vi "iRobot Poll Sensor Group 4.vi"(8 "error in":errorcluster, 11 "UART port in":T4) -> (0 "error out":errorcluster, 1 "Timed Out?":bool, 2 "Sensor Group 4":T1, 3 "UART port out":T4)   [LabVIEW 2010]
doc: "Poll the iRobot for Sensor Group 4; blocks until response is received, or the operation has timed out.\n\nThis VI both writes to AND reads from the serial port\n<b>NOTE</b>: This should not be used in a loop if other serial reading or writing VIs are called in parallel loops."
uses:
  UART/UART Port Type.ctl
  Sensor Controls/iRobot Sensor Group 4.ctl
  Sensor Controls/iRobot Cargo Bay Digital Inputs.ctl
  Sensor Controls/iRobot Charging Sources Available.ctl
  Open Interface Controls/iRobot Sensor ID.ctl
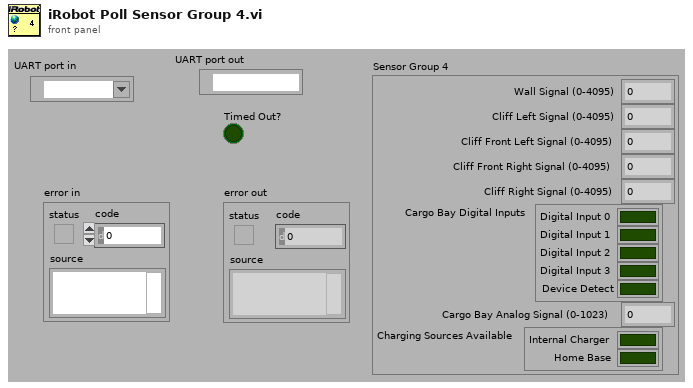
[diagram p1: front panel]
types:
  T1 = typedef "iRobot Sensor Group 4.ctl" = cluster{"Wall Signal (0-4095)":u16, "Cliff Left Signal (0-4095)":u16, "Cliff Front Left Signal (0-4095)":u16, "Cliff Front Right Signal (0-4095)":u16, "Cliff Right Signal (0-4095)":u16, "Cargo Bay Digital Inputs":T2, "Cargo Bay Analog Signal (0-1023)":u16, "Charging Sources Available":T3}
  T2 = typedef "iRobot Cargo Bay Digital Inputs.ctl" = cluster{"Digital Input 0":bool, "Digital Input 1":bool, "Digital Input 2":bool, "Digital Input 3":bool, "Device Detect":bool}
  T3 = typedef "iRobot Charging Sources Available.ctl" = cluster{"Internal Charger":bool, "Home Base":bool}
  T4 = typedef "UART Port Type.ctl" = refnum<visa-resource-name>
  T5 = typedef "iRobot Sensor ID.ctl" = enum8{"Sensor Group 0", "Sensor Group 1", "Sensor Group 2", "Sensor Group 3", "Sensor Group 4", "Sensor Group 5", "Sensor Group 6", "Bump + Wheel Drop", "Wall", "Cliff Left", "Cliff Front Left", "Cliff Front Right", "Cliff Right", "Virtual Wall", "Low Side Driver + Wheel Overcurrent", "Unused 0", "Unused 1", "Infrared", "Buttons", "Distance", "Angle", "Charging State", "Voltage", "Current", "Battery Temperature", "Battery Charge", "Battery Capacity", "Wall Signal", "Cliff Left Signal", "Cliff Front Left Signal", "Cliff Front Right Signal", "Cliff Right Signal", "Cargo Bay Digital Inputs", "Cargo Bay Analog Signal", "Charging Sources Available", "OI Mode", "Song Number", "Song Playing", "Number of Stream Packets", "Requested Velocity", "Requested Radius", "Requested Right Velocity", "Requested Left Velocity"}
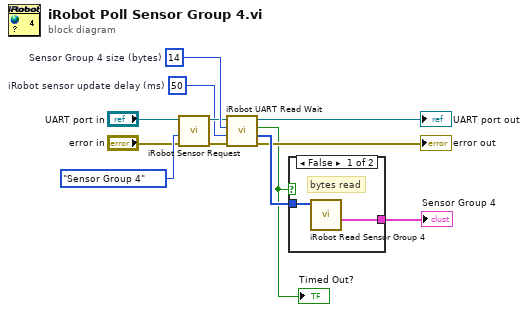
[diagram p0: block diagram]
diagram:
  w3 = 50  # iRobot sensor update delay (ms)
  w11 = 14  # Sensor Group 4 size (bytes)
  n1 = call "iRobot Sensor Request.vi"("error in"="error in", "Sensor ID"=iRobot_Sensor_ID."Sensor Group 4", "UART port in"="UART port in") -> ("error out"=w6:errorcluster, "UART port out"=w9:T4)  [unwired: 7 in]
  n2 = call "iRobot UART Read Wait.vi"("error in"=w6, "timeout (ms)"=w3, "Number of Bytes"=w11, "UART port in"=w9) -> ("error out"=→"error out":errorcluster, "UART Stream"=w10:u8[], "Timed Out?"=w2:bool, "UART port out"=→"UART port out":T4)  [unwired: 4 in]
  "Timed Out?" <- w2
  n3 = case shown="False" w2 {
    tunnel: w10 -> [w14 _]
    tunnel: [w13 _] -> w1
    frame False {
      # "bytes read"
      n4 = call "iRobot Read Sensor Group 4.vi"("stream in"=w14) -> ("Sensor Group 4"=w13:T1)  [unwired: 9 in, 1 out]
    }
    frame True {
      # "timeout"
    }
  }
  "Sensor Group 4" <- w1
